vi "TestExec.Factory Logix UUT Step Check, Use DB Stored Procedure_In WOrk.vi"(8 "error in (no error)":errorcluster, 9 "SN":string, 11 "UDL File":path) -> (0 "error out":errorcluster, 3 "Results":string[][](table))   [LabVIEW 2018]
doc: "This VI calls stored procedures in SQL Server using the LabVIEW Database Connectivity Toolset. The VI uses two methods to call the built-in stored procedure sp_helpuser -- one method uses parameters and the other does not."
uses:
  <vilib>/addons/database/Auxilliary.llb/DB Tools Parameter Info.ctl
  <vilib>/addons/database/Auxilliary.llb/DB Tools DataTypes.ctl
  <vilib>/addons/database/Auxilliary.llb/DB Tools Parameter Dir.ctl
  <vilib>/addons/database/Connection.llb/DB Tools Open Connec (Path).vi
  <vilib>/addons/database/Command.llb/Cmd Set Parameter Value (C).vi
  <vilib>/addons/database/Command.llb/Cmd Execute.vi
  <vilib>/addons/database/Recordset.llb/Rec Fetch Recordset Data (CR).vi
  <vilib>/addons/database/Recordset.llb/Rec Destroy - Command.vi
  <vilib>/addons/database/Command.llb/Cmd Delete.vi
  <vilib>/addons/database/Connection.llb/Conn Execute.vi
  <vilib>/addons/database/Recordset.llb/Rec Fetch Recordset Data (R).vi
  <vilib>/addons/database/Recordset.llb/Rec Destroy - Connection.vi
  <vilib>/addons/database/_DB Variant To Data/Database Variant To Data.xnode
  <vilib>/addons/database/NI_Database_API.lvlib
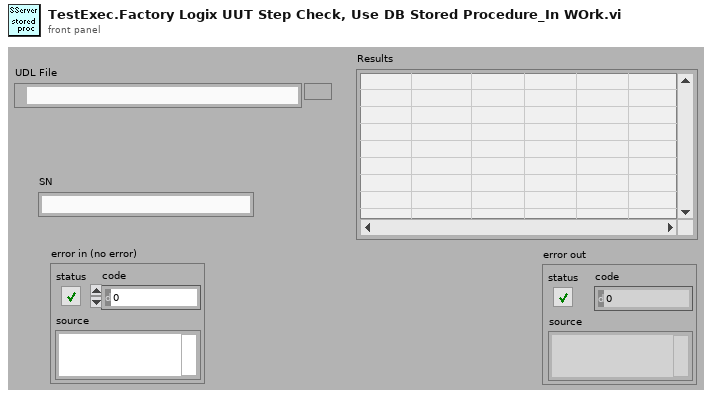
[diagram p1: front panel]
types:
  T1 = typedef "NI_Database_API.lvlib/Conn ObjectReference.ctl" = refnum<k1>
  T2 = typedef "NI_Database_API.lvlib/DB Tools Parameter Info.ctl" = cluster{"parameter name":string, "type":T3, "direction":T4, "value":variant}
  T3 = typedef "NI_Database_API.lvlib/DB Tools DataTypes.ctl" = enum16{"String", "Long (I32)", "Single (SGL)", "Double (DBL)", "Date/Time", "Binary"}
  T4 = typedef "NI_Database_API.lvlib/DB Tools Parameter Dir.ctl" = enum32{"Input", "Output", "Input/Output", "Return Value"}
  T5 = typedef "NI_Database_API.lvlib/Cmd ObjectReference.ctl" = refnum<k1>
  T6 = typedef "NI_Database_API.lvlib/Cmd-Rec Object Reference.ctl" = refnum<k1>
  T7 = typedef "NI_Database_API.lvlib/Rec ObjectReference.ctl" = refnum<k1>
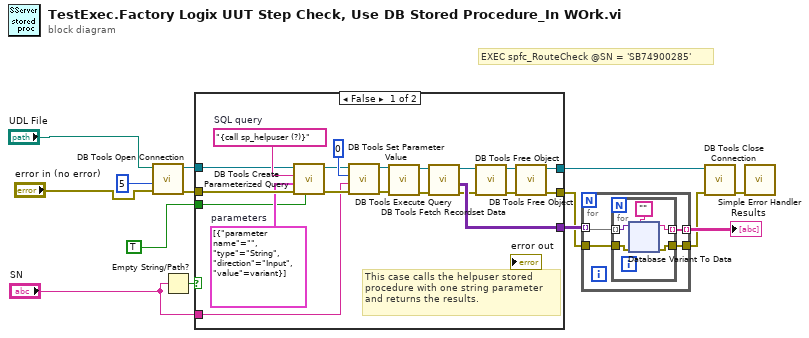
[diagram p0: block diagram]
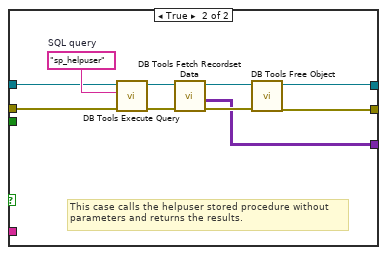
[diagram p2: hidden frame]
diagram:
  # "EXEC spfc_RouteCheck @SN = 'SB74900285'"
  n1 = call-poly <vilib>:"DB Tools Open Connection.vi"("error in (no error)"="error in (no error)", "connection timeout (15)"=5, "connection information"="UDL File") -> ("error out"=w14:errorcluster, "connection reference"=w13:T1)  [unwired: 5 in]
  n2 = Empty String/Path?(string/path="SN") -> (empty?=w8:bool)
  n3 = case shown="False" w8 {
    tunnel: w14 -> [w28 w42]
    tunnel: w13 -> [w27 w43]
    tunnel: [w16 w38] -> w5
    tunnel: [w15 w37] -> w7
    tunnel: TRUE ("stored procedure?") -> [w25 _]
    tunnel: "SN" -> [w22 _]
    tunnel: [w20 w35] -> w9
    frame False {
      w26 = T2[] [{"parameter name"="", "type"=enum."String", "direction"=enum."Input", "value"=variant}]  # parameters
      w29 = "{call sp_helpuser (?)}"  # SQL query
      # "This case calls the helpuser stored\nprocedure with one string parameter \nand returns the results."
      n4 = call <vilib>:"DB Tools Create Parameterized Query.vi"("stored procedure? (F)"=w25, "error in (no error)"=w28, "parameters"=w26, "SQL query"=w29, "connection reference"=w27) -> ("error out"=w32:errorcluster, "command reference"=w30:T5)  [unwired: 2 in, 1 out]
      n5 = call-poly <vilib>:"DB Tools Set Parameter Value.vi"("error in (no error)"=w32, "value"=w22, "parameter index"=0, "command reference"=w30) -> ("error out"=w33:errorcluster, "command reference out"=w34:T5)  [unwired: 4 in]
      n6 = call-poly <vilib>:"DB Tools Execute Query.vi"("error in (no error)"=w33, "command reference"=w34) -> ("error out"=w24:errorcluster, "command-recordset reference"=w23:T6)  [unwired: 6 in]
      n7 = call-poly <vilib>:"DB Tools Fetch Recordset Data.vi"("error in (no error)"=w24, "command-recordset reference"=w23) -> ("error out"=w19:errorcluster, "recordset data"=w20:variant[][], "command-recordset reference out"=w21:T6)  [unwired: 3 in]
      n8 = call-poly <vilib>:"DB Tools Free Object.vi"("error in (no error)"=w19, "command-recordset reference"=w21) -> ("error out"=w17:errorcluster, "command reference"=w18:T5)  [unwired: 8 in]
      n9 = call-poly <vilib>:"DB Tools Free Object.vi"("error in (no error)"=w17, "command reference"=w18) -> ("error out"=w15:errorcluster, "connection reference"=w16:T1)  [unwired: 8 in]
    }
    frame True {
      w44 = "sp_helpuser"  # SQL query
      # "This case calls the helpuser stored procedure without\nparameters and returns the results."
      n10 = call-poly <vilib>:"DB Tools Execute Query.vi"("error in (no error)"=w42, "SQL query"=w44, "connection reference"=w43) -> ("error out"=w40:errorcluster, "recordset reference"=w41:T7)  [unwired: 5 in]
      n11 = call-poly <vilib>:"DB Tools Fetch Recordset Data.vi"("error in (no error)"=w40, "recordset reference"=w41) -> ("error out"=w36:errorcluster, "recordset data"=w35:variant[][], "recordset reference out"=w39:T7)  [unwired: 3 in]
      n12 = call-poly <vilib>:"DB Tools Free Object.vi"("error in (no error)"=w36, "recordset reference"=w39) -> ("error out"=w37:errorcluster, "connection reference"=w38:T1)  [unwired: 8 in]
    }
  }
  n13 = for {
    tunnel: [w48] -> w10 mode=indexing
    tunnel: w9 -> [w47] mode=indexing
    tunnel: w7 -> [w46]
    tunnel: [w45] -> w6
    n14 = for {
      tunnel: [w52] -> w48 mode=indexing
      tunnel: w47 -> [w51] mode=indexing
      tunnel: w46 -> [w50]
      tunnel: [w49] -> w45
      n15 = xnode "Database Variant To Data"("database variant"=w51, "error in (no error)"=w50, "type"="") -> ("data"=w52:string, "error out"=w49:errorcluster)
    }
  }
  "Results" <- w10
  n16 = call <vilib>:"DB Tools Close Connection.vi"("error in (no error)"=w6, "connection reference"=w5) -> ("error out"=w12:errorcluster)  [unwired: 5 in]
  n17 = call <vilib>:"Simple Error Handler.vi"("error in (no error)"=w12) -> ()  [unwired: 4 in, 5 out]
